vi "Create_Trajectories.vi"(8 "error in":errorcluster caption="entrée d'erreur", 11 "Type of pattern":T1(ring)=enum."spiralScan") -> (0 "error out":errorcluster caption="sortie d'erreur", 2 "Trajectories":cluster{dbl[], dbl[]}(graph), 3 "Trajectories":dbl[][](graph))   [LabVIEW 2025]
panel:
  out "données":i32
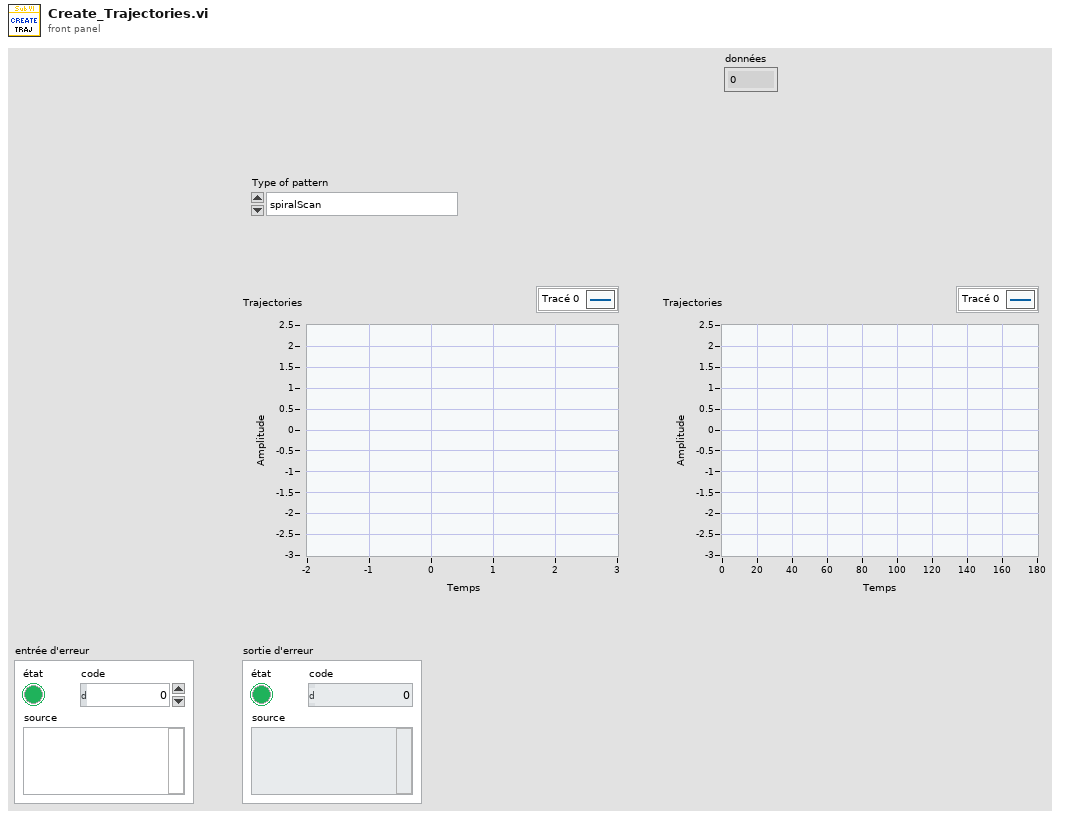
[diagram p1: front panel]
types:
  T1 = enum16{"rasterScan", "snakeMovement", "circularScan", "circularTIR", "spiralScan"}
  T2 = enum16{"big-endian, network order", "native, host order", "little-endian"}
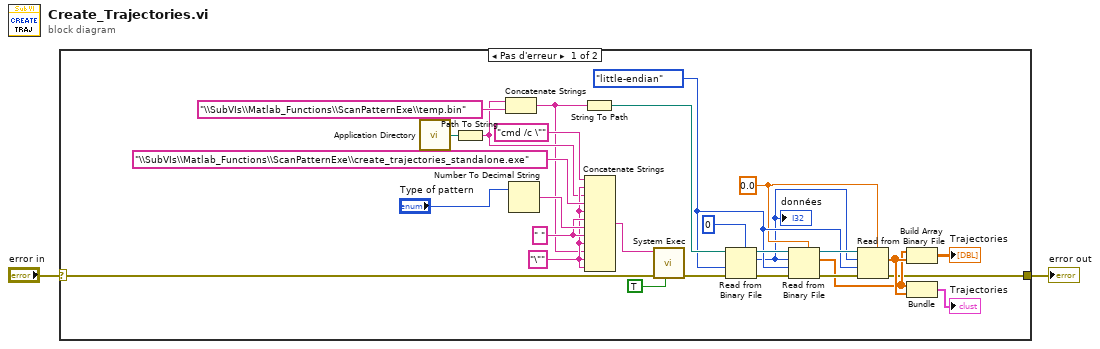
[diagram p0: block diagram]
diagram:
  n1 = case shown="Pas d'erreur" "error in" {
    selector: "error in" -> [w4 w31]
    tunnel: [w3 w31] -> w1
    frame No Error {
      w9 = 0.0
      w11 = T2."little-endian" ("ordre des octets (0 : big-Endian, network order)")
      w25 = " " ("chaîne")
      w22 = "\"" ("chaîne")
      n2 = call <vilib>:"Application Directory.vi"() -> ("Application Directory"=w28:path)
      n3 = Path To String(path=w28) -> (string=w20:string)
      n4 = Concatenate Strings(w20, "\\SubVIs\\Matlab_Functions\\ScanPatternExe\\temp.bin" ("chaîne")) -> (w19:string)
      n5 = Number To Decimal String(number="Type of pattern") -> (decimal integer string=w26:string)  [unwired: 1 in]
      n6 = String To Path(string=w19) -> (path=w18:path)
      n7 = Concatenate Strings("cmd /c \"" ("chaîne"), w22, w20, "\\SubVIs\\Matlab_Functions\\ScanPatternExe\\create_trajectories_standalone.exe" ("chaîne"), w22, w25, w26, w25, w22, w19, w22, w22) -> (w24:string)
      n8 = call <vilib>:"System Exec.vi"("run minimized? (F)"=TRUE, "error in (no error)"=w4, "command line"=w24) -> ("error out"=w16:errorcluster)  [unwired: 5 in, 3 out]
      n9 = Read from Binary File(5:0, 8:w16, 9:w11, 11:w18) -> (0:w17:errorcluster, 2:w8:i32, 3:w15:refnum<file>)  [unwired: 2 in, 1 out]
      "données" <- w8
      n10 = Read from Binary File(5:w9, 8:w17, 9:w11, 10:w8, 11:w15) -> (0:w13:errorcluster, 2:w7:dbl[], 3:w14:refnum<file>)  [unwired: 1 in, 1 out]
      n11 = Read from Binary File(5:w9, 8:w13, 9:w11, 10:w8, 11:w14) -> (0:w3:errorcluster, 2:w10:dbl[])  [unwired: 1 in, 2 out]
      n12 = Build Array(w7, w10) -> (→"Trajectories":dbl[][])
      n13 = Bundle(w7, w10) -> (→"Trajectories":cluster{dbl[], dbl[]})  [unwired: 1 in]
    }
    frame Error {
    }
  }
  "error out" <- w1
